vi "table name alarms.vi"(3 "object name":string) -> (0 "table name trunc":string, 1 "table name curr":string)   [LabVIEW 2019]
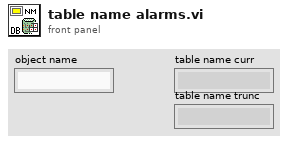
[diagram p1: front panel]
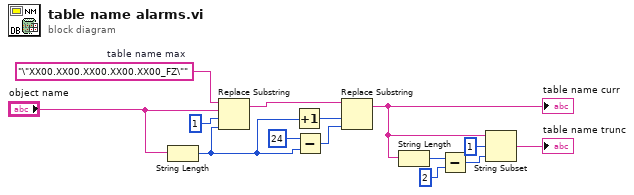
[diagram p0: block diagram]
diagram:
  w13 = "\"XX00.XX00.XX00.XX00.XX00_FZ\""  # table name max
  n1 = String Length(string="object name") -> (length=w11:i32)
  n2 = Replace Substring(2:w11, 3:1 ("offset (0)"), 4:"object name", 5:w13) -> (1:w1:string)  [unwired: 1 out]
  n3 = Increment(x=w11) -> (x+1=w14:i32)
  n4 = Subtract(x=24 ("length (len. of substring)"), y=w11) -> (x-y=w12:i32)
  n5 = Replace Substring(2:w12, 3:w14, 5:w1) -> (1:w3:string)  [unwired: 1 in, 1 out]
  "table name curr" <- w3
  n6 = String Length(string=w3) -> (length=w5:i32)
  n7 = Subtract(x=w5, y=2) -> (x-y=w6:i32)
  n8 = String Subset(string=w3, offset (0)=1, length (rest)=w6) -> (substring=→"table name trunc":string)
